vi "_unitOperForRS232_EEPROM_vna_jet.vi"(0 "Operations":string(combo)="read data", 1 "Data to write":u8[](array[numeric])=[46, 46, 46, 46, 46, 46, 46, 76, 117, 120, 115, 104, 97, 114, 101, 32, 83, 90, 32, 32, 32, 32, 32, 32, 0, 0, 9, 58, 88, 88, 88, 88, 88, 45, 88, 88, 88, 88, 32, 32, 32, 32, 32, 32, 69, 32, 32, 32, 0, 0, 0, 0, 0, 56, 56, 56, 56, 56, 56, 56, 56, 56, 56, 32, 32, 32, 32, 32, 32, 48, 56, 48, 51, 51, 0, 0, 0, 0, 0, 46, 46, 46, 46, 46, 46, 46, 46, 46, 46, 32, 105, 50, 99, 32, 116, 101, 115, 116, 105, 110, 103, 45, 45, 45, 45, 45, 32, 99, 111, 109, 112, 108, 101, 116, 101, 100, 32, 97, 110, 100, 32, 115, 117, 99, 99, 101, 115, 115, 102, 117, 108] format="%x", 3 "StartByte":i32 format="%.0x", 6 "Steps":string[](array[string])=["modify byte 127", "read byte 0 to 127", "read byte 128 to 255"], 7 "W&RDLength":i32=86, 12 "Auto":bool=TRUE) -> (15 "random_array":i32[](array[numeric])=[255, 255, 0, 0, 0, 0, 0, 0, 0, 0, 0, 0, 0, 0, 0, 0, 0, 0, 0, 0, 0, 0, 0, 0, 0, 0, 0, 0, 0, 0, 0, 0] format="%.0x", 17 "Message":string="Read EEPROM", 19 "R A I 128 to 255":u8[](array[numeric])=[3, 4, 33, 1, 0, 0, 4, 65, 132, 128, 213, 0, 103, 0, 0, 0, 0, 0, 1, 0, 72, 73, 83, 69, 84, 69, 67, 0, 0, 0, 0, 0, 0, 0, 0, 0, 0, 0, 0, 0, 76, 48, 48, 84, 72, 48, 48, 50, 45, 77, 49, 45, 82, 0, 0, 0, 65, 0, 0, 0, 1, 0, 0, 250, 0, 0, 0, 0, 49, 50, 51, 50, 55, 49, 48, 48, 48, 51, 0, 0, 0, 0, 0, 0, 49, 50, 49, 49, 50, 50, 0, 0, 0, 0, 0, 28, 72, 51, 67, 0, 0, 0, 0, 0, 0, 0, 0, 48, 52, 48, 52, 65, 49, 49, 50, 1, 2, 0, 1, 0, 0, 0, 0, 0, 0, 0, 0, 95, 0, 0, 0, 0, 0, 0, 0, 0, 0, 0, 0, 0, 0, 0, 0, 0, 0, 0, 0, 0, 0, 0, 0, 0, 0, 0, 0, 0, 0, 0, 0, 0, 0, 0, 0, 0, 0, 0, 0, 0, 0, 0, 0, 0, 0, 0, 0, 0, 0, 0, 0, 0, 0, 0, 0, 0, 0, 0, 0, 0, 0, 0, 0, 0, 0, 0, 0, 0, 0, 0, 0, 0, 0, 0, 0, 0, 0, 0, 0, 0, 0, 0, 0, 0, 0, 0, 0, 0, 0, 0, 0, 0, 0, 0, 0, 0, 0, 0, 0, 0, 0, 0, 0, 0, 0, 0, 0, 0, 0, 0, 0, 0, 0, 0, 0, 0, 0, 0, 0, 0, 0, 0, 0, 0, 0, 0, 0, 0] format="%x")   [LabVIEW 2011]
panel:
  in  "Commands_input":string[](array[string])
  out "rad_num":string
  out "EndByte":i32=86
  out "RD A 128 to 255":string[][](array[string])
  out "RD 128 to 255":string
  in  "WData size":u32=1
  out "Result":bool=TRUE
  out "VISA resource":refnum<visa-resource-name>="COM1"
  out "error out":errorcluster={"status"=FALSE, "code"=1073676294, "source"="RS232-I2C-EEPROM.vi中的VISA读取"}
  in  "VISA resource name":refnum<visa-resource-name>="COM1"
  in  "Select channel":u32 max=1
  in  "Mode":u32(ring) items=["0~EasyI2C", "1~TimingI2C"]
  # "1"
  # "2"
  # "3"
  # "序号       0 to 127  128 to 255"
  # "0 to 127  128 to 255"
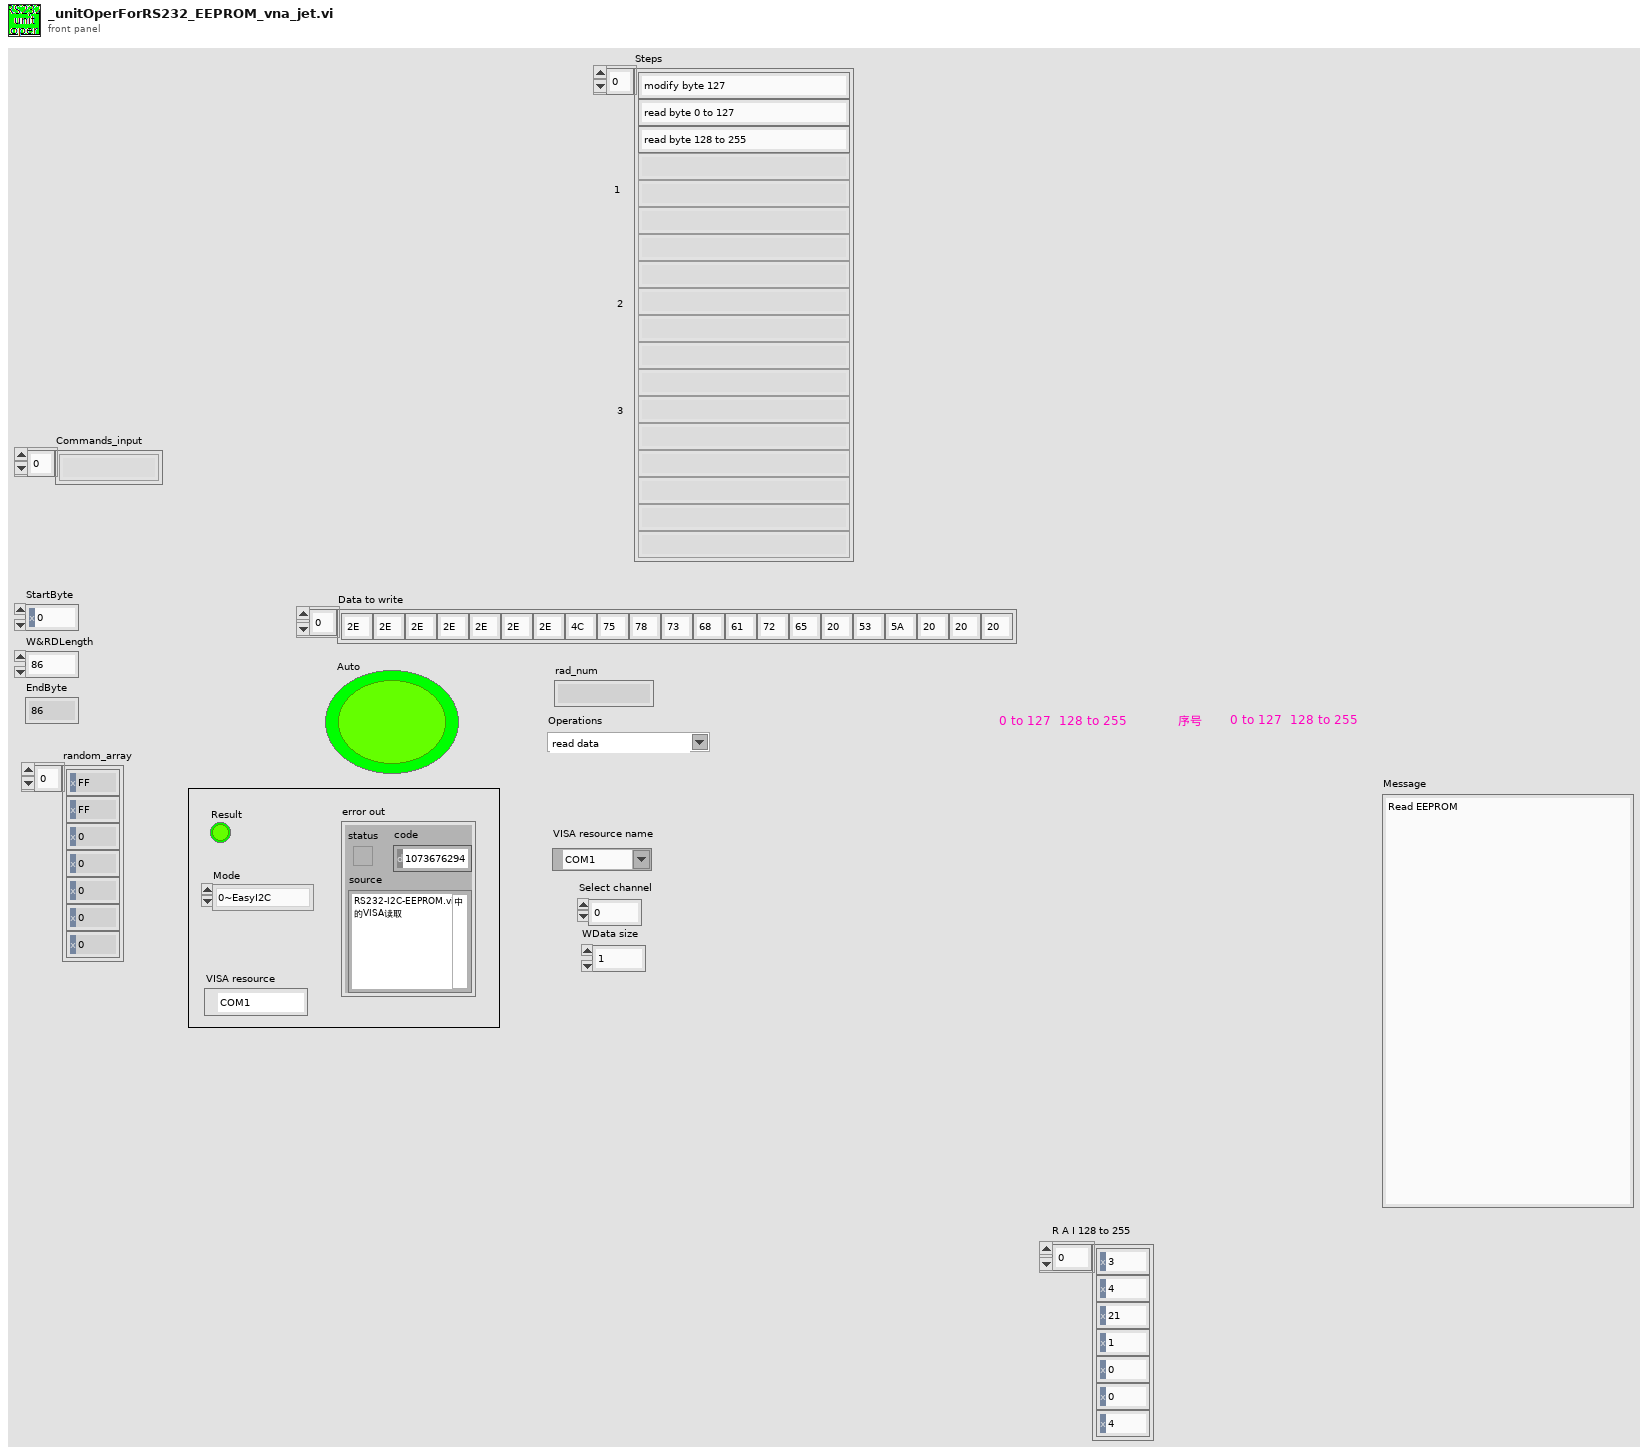
[diagram p1: front panel]
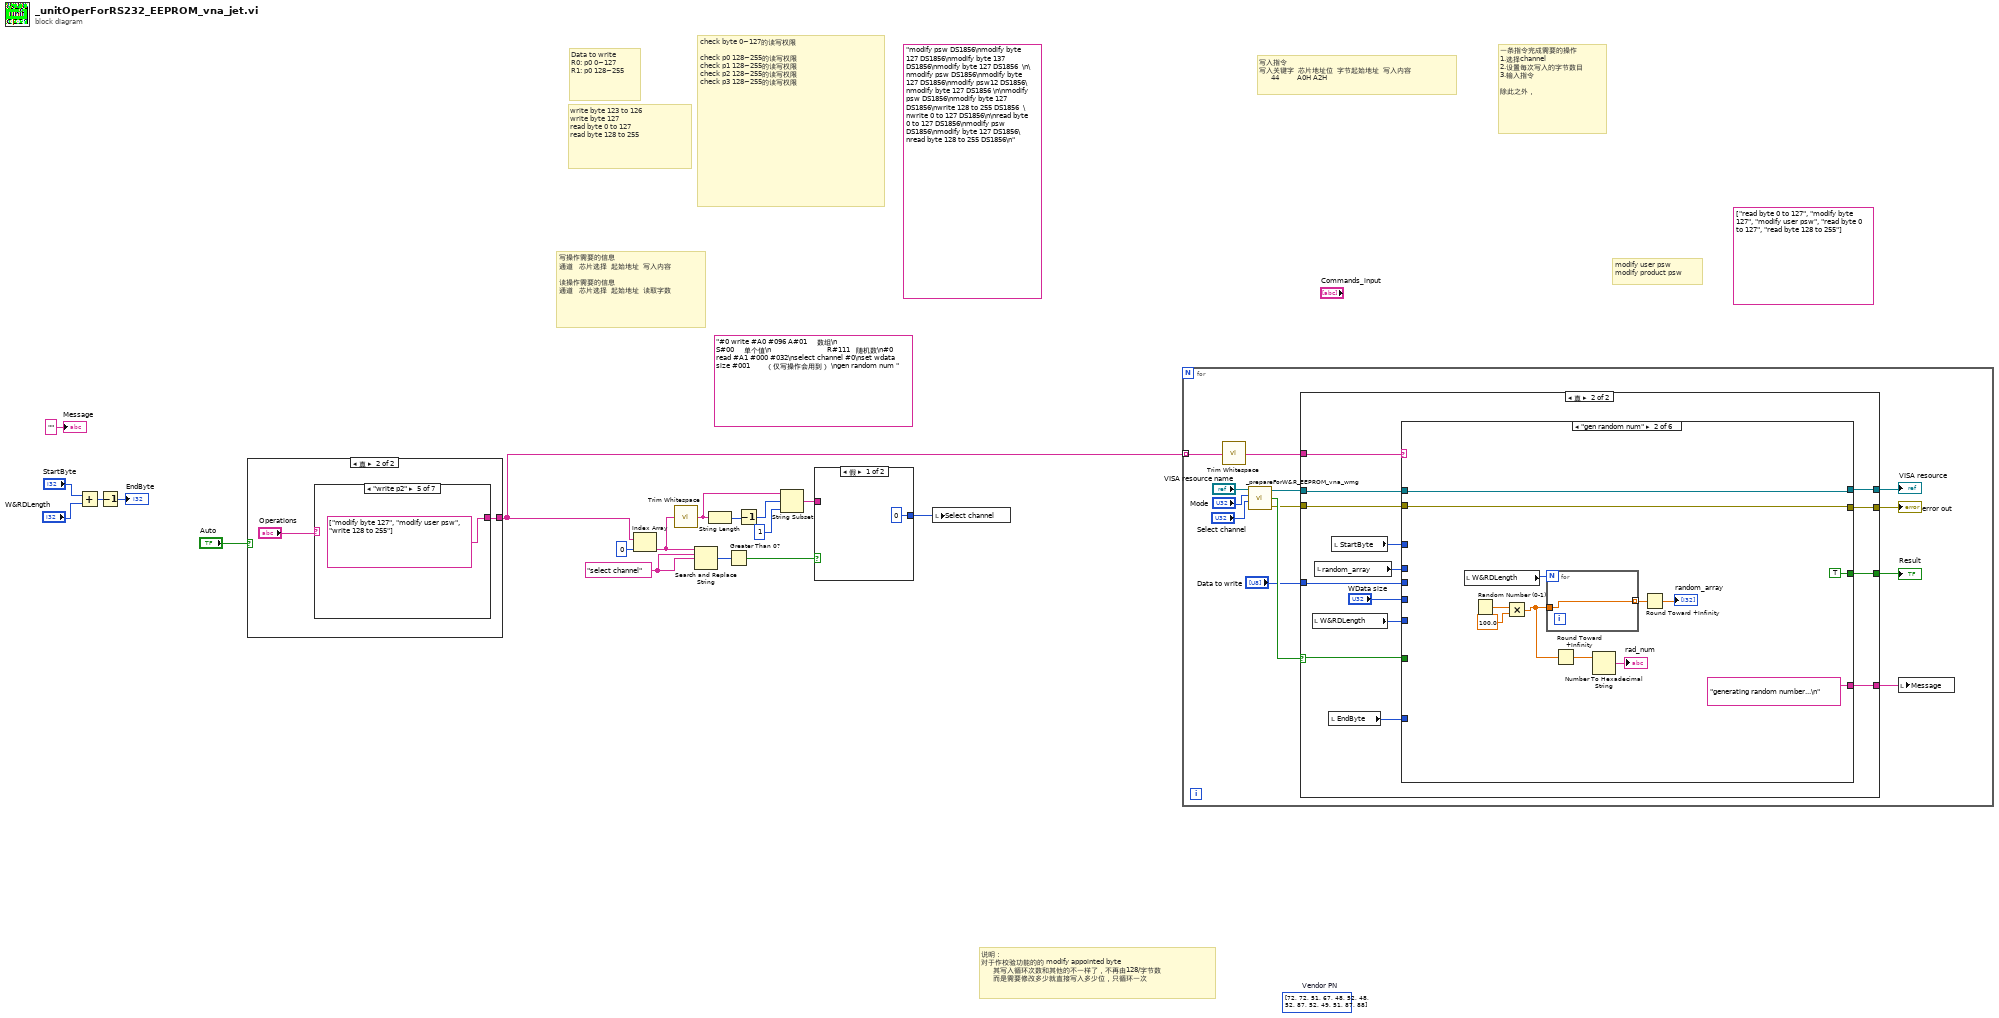
[diagram p0: block diagram]
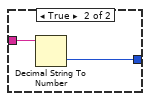
[diagram p2: hidden frame]
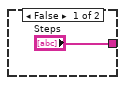
[diagram p3: hidden frame]
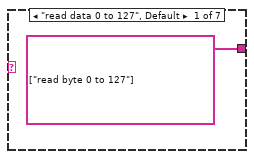
[diagram p4: hidden frame]
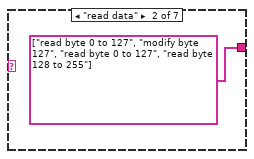
[diagram p5: hidden frame]
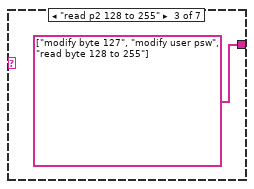
[diagram p6: hidden frame]
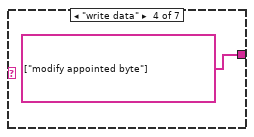
[diagram p7: hidden frame]
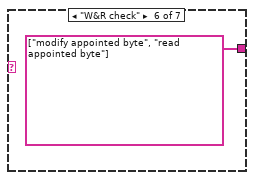
[diagram p8: hidden frame]
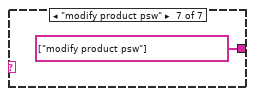
[diagram p9: hidden frame]
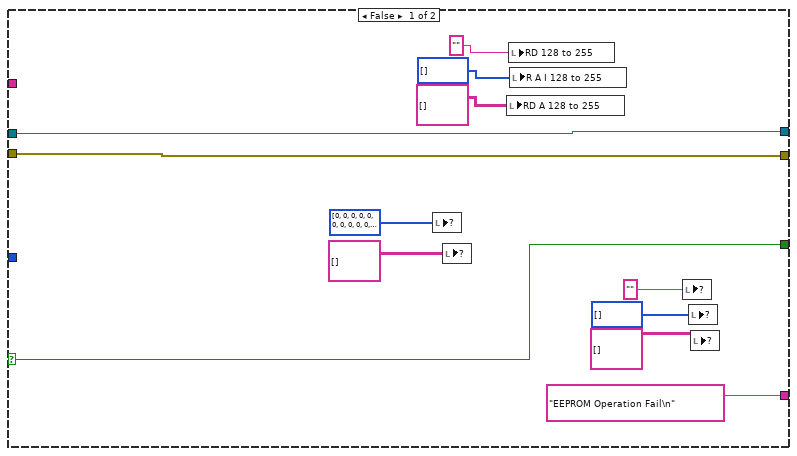
[diagram p10: hidden frame]
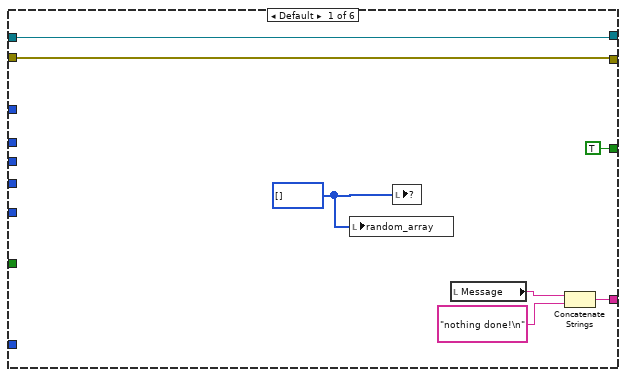
[diagram p11: hidden frame]
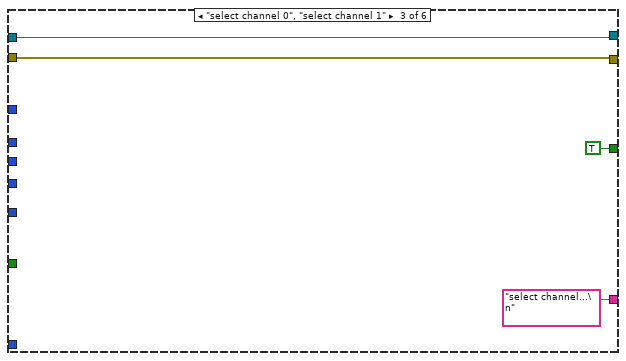
[diagram p12: hidden frame]
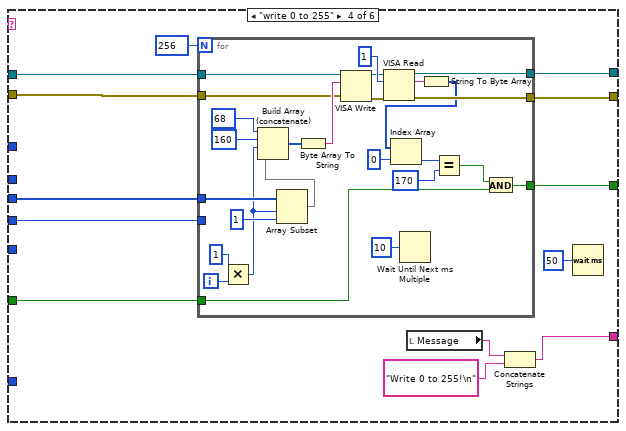
[diagram p13: hidden frame]
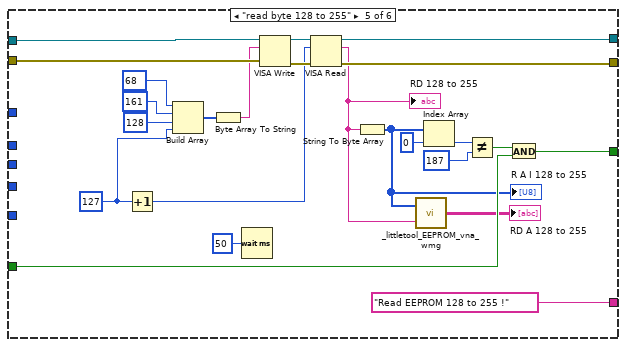
[diagram p14: hidden frame]
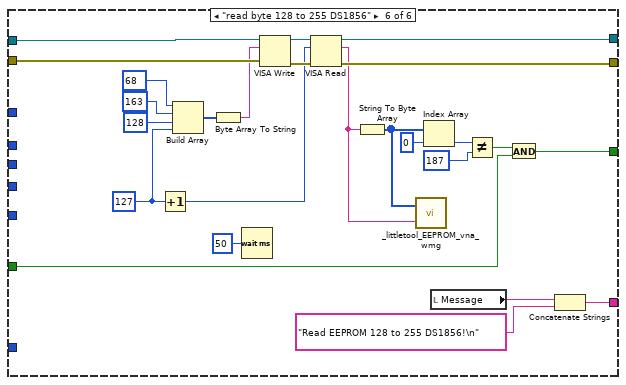
[diagram p15: hidden frame]
diagram:
  w10 = "select channel" ("搜索字符串")
  (unwired) i32[] [72, 72, 51, 67, 48, 52, 48, 52, 87, 52, 49, 51, 87, 88]  # Vendor PN
  (unwired) string[] ["read byte 0 to 127", "modify byte 127", "modify user psw", "read byte 0 to 127", "read byte 128 to 255"]
  (unwired) "#0 write #A0 #096 A#01     数组\n                            S#00     单个值\n                            R#111   随机数\n#0 read #A1 #000 #032\nselect channel #0\nset wdata size #001        （仅写操作会用到） \ngen random num "
  (unwired) "modify psw DS1856\nmodify byte 127 DS1856\nmodify byte 137 DS1856\nmodify byte 127 DS1856  \n\nmodify psw DS1856\nmodify byte 127 DS1856\nmodify psw12 DS1856\nmodify byte 127 DS1856 \n\nmodify psw DS1856\nmodify byte 127 DS1856\nwrite 128 to 255 DS1856  \nwrite 0 to 127 DS1856\n\nread byte 0 to 127 DS1856\nmodify psw DS1856\nmodify byte 127 DS1856\nread byte 128 to 255 DS1856\n"
  # "说明：\n对于作校验功能的的 modify appointed byte\n      其写入循环次数和其他的不一样了，不再由128/字节数\n      而是需要修改多少就直接写入多少位，只循环一次"
  # "写操作需要的信息\n通道   芯片选择  起始地址  写入内容\n\n读操作需要的信息\n通道   芯片选择  起始地址  读取字数"
  # "一条指令完成需要的操作\n1.选择channel\n2.设置每次写入的字节数目\n3.输入指令\n\n除此之外，"
  # "写入指令\n写入关键字  芯片地址位  字节起始地址  写入内容\n      44         A0H A2H"
  # "modify user psw\nmodify product psw"
  # "check byte 0~127的读写权限\n      \ncheck p0 128~255的读写权限\ncheck p1 128~255的读写权限\ncheck p2 128~255的读写权限\ncheck p3 128~255的读写权限"
  # "Data to write\nR0: p0 0~127\nR1: p0 128~255"
  # "write byte 123 to 126\nwrite byte 127\nread byte 0 to 127\nread byte 128 to 255"
  n1 = Add(x="StartByte", y="W&RDLength") -> (x+y=w14:i32)
  n2 = Decrement(x=w14) -> (x-1=→"EndByte":i32)
  n3 = case shown="真" "Auto" {
    tunnel: ["Steps" w21] -> w18
    frame False {
    }
    frame True {
      n4 = case shown="\"write p2\"" "Operations" {
        tunnel: [string[] ["read byte 0 to 127"] string[] ["read byte 0 to 127", "modify byte 127", "read byte 0 to 127", "read byte 128 to 255"] string[] ["modify byte 127", "modify user psw", "read byte 128 to 255"] string[] ["modify appointed byte"] string[] ["modify byte 127", "modify user psw", "write 128 to 255"] string[] ["modify appointed byte", "read appointed byte"] string[] ["modify product psw"]] -> w21
        frame "read data 0 to 127", Default {
        }
        frame "read data" {
        }
        frame "read p2 128 to 255" {
        }
        frame "write data" {
        }
        frame "write p2" {
        }
        frame "W&R check" {
        }
        frame "modify product psw" {
        }
      }
    }
  }
  n5 = Index Array(array=w18, index=0 ("索引")) -> (element=w7:string)
  n6 = call <vilib>:"Trim Whitespace.vi"("string"=w7) -> ("trimmed string"=w6:string)  [unwired: 1 in]
  n7 = Search and Replace String(input string=w7, search string=w10, replace string=w10) -> (number of replacements=w9:i32)  [unwired: 5 in, 3 out]
  n8 = String Length(string=w6) -> (length=w5:i32)
  n9 = Greater Than 0?(x=w9) -> (x > 0?=w8:bool)
  n10 = Decrement(x=w5) -> (x-1=w4:i32)
  n11 = String Subset(string=w6, offset (0)=w4, length (rest)=1 ("长度（剩余）")) -> (substring=w2:string)
  n12 = case shown="假" w8 {
    tunnel: w2 -> [_ w31]
    tunnel: [0 w30] -> w1
    frame False {
    }
    frame True {
      n13 = Decimal String To Number(string=w31) -> (number=w30:i32)  [unwired: 2 in, 1 out]
    }
  }
  n14 = local write "Select channel"(w1) -> ()
  n15 = for {
    tunnel: w18 -> [w33] mode=indexing
    n16 = call <vilib>:"Trim Whitespace.vi"("string"=w33) -> ("trimmed string"=w32:string)  [unwired: 1 in]
    n17 = call "_prepareForW&R_EEPROM_vna_wmg.vi"("Select channel"="Select channel", "Mode"="Mode", "VISA resource name"="VISA resource name") -> ("错误输出"=w41:errorcluster, "x = y?"=w44:bool, "VISA资源名称输出"=w43:refnum<visa-resource-name>)  [unwired: 1 in]
    n18 = case shown="真" w44 {
      selector: w44 -> [w53 w65]
      tunnel: w43 -> [w55 w70]
      tunnel: w41 -> [w56 w69]
      tunnel: w32 -> [_ w68]
      tunnel: "Data to write" -> [_ w67]
      tunnel: [w56 w64] -> w36
      tunnel: [w55 w63] -> w37
      tunnel: ["EEPROM Operation Fail\n" ("message") w62] -> w35
      tunnel: [w53 w61] -> w34
      frame False {
        n19 = local write item#-1(i32[] [0, 0, 0, 0, 0, 0, 0, 0, 0, 0, 0, 0, 0, 0, 0, 0, 0, 0, 0, 0, 0, 0, 0, 0, 0, 0, 0, 0, 0, 0, 0, 0, 0, 0, 0, 0, 0, 0, 0, 0, 0, 0, 0, 0, 0, 0, 0, 0, 0, 0, 0, 0, 0, 0, 0, 0, 0, 0, 0, 0, 0, 0, 0, 0, 0, 0, 0, 0, 0, 0, 0, 0, 0, 0, 0, 0, 0, 0, 0, 0, 0, 0, 0, 0, 0, 0, 0, 0, 0, 0, 0, 0, 0, 0, 0, 0, 0, 0, 0, 0, 0, 0, 0, 0, 0, 0, 0, 0, 0, 0, 0, 0, 0, 0, 0, 0, 0, 0, 0, 0, 0, 0, 0, 0, 0, 0, 0, 0, 0, 0, 0, 0, 0, 0, 0, 0, 0, 0, 0, 0, 0, 0, 0, 0, 0, 0, 0, 0, 0, 0, 0, 0, 0, 0, 0, 0, 0, 0, 0, 0, 0, 0, 0, 0, 0, 0, 0, 0, 0, 0, 0, 0, 0, 0, 0, 0, 0, 0, 0, 0, 0, 0, 0, 0, 0, 0, 0, 0, 0, 0, 0, 0, 0, 0, 0, 0, 0, 0, 0, 0, 0, 0, 0, 0, 0, 0, 0, 0, 0, 0, 0, 0, 0, 0, 0, 0, 0, 0, 0, 0, 0, 0, 0, 0, 0, 0, 0, 0, 0, 0, 0, 0, 0, 0, 0, 0, 0, 0, 0, 0, 0, 0, 0, 0, 0, 0, 0, 0, 0, 0, 0, 0, 0, 0, 0, 0] ("Data from Read")) -> ()
        n20 = local write item#-1(string[][] [] ("EEPROM read data")) -> ()
        n21 = local write "RD A 128 to 255"(string[][] [] ("R A C 0 to 127")) -> ()
        n22 = local write "RD 128 to 255"("") -> ()
        n23 = local write "R A I 128 to 255"(u8[] [] ("R A I 0 to 127")) -> ()
        n24 = local write item#-1("") -> ()
        n25 = local write item#-1(u8[] [] ("R A I 0 to 127")) -> ()
        n26 = local write item#-1(string[][] [] ("R A C 0 to 127")) -> ()
      }
      frame True {
        n27 = local read "W&RDLength"() -> (w58:i32)
        n28 = local read "random_array"() -> (w59:i32[])
        n29 = local read "EndByte"() -> (w57:i32)
        n30 = local read "StartByte"() -> (w60:i32)
        n31 = case shown="\"gen random num\"" w68 {
          tunnel: w70 -> [w77 w88 w94 w107 w157 w182]
          tunnel: w69 -> [w75 w87 w93 w106 w156 w181]
          tunnel: w67 -> [_ _ _ w100 _ _]
          tunnel: [w77 w88 w94 w103 w151 w176] -> w63
          tunnel: [w75 w87 w93 w105 w150 w175] -> w64
          tunnel: "WData size" -> [_ _ _ w104 _ _]
          tunnel: w65 -> [_ _ _ w102 w145 w171]
          tunnel: [w73 "generating random number...\n" ("Message") "select channel...\n" ("Message") w95 "Read EEPROM 128 to 255 !" ("Message") w161] -> w62
          tunnel: [TRUE TRUE TRUE w101 w143 w169] -> w61
          tunnel: w60 -> [_ _ _ _ _ _]
          tunnel: w59 -> [_ _ _ _ _ _]
          tunnel: w58 -> [_ _ _ _ _ _]
          tunnel: w57 -> [_ _ _ _ _ _]
          frame Default {
            w74 = i32[] []
            n32 = local write "random_array"(w74) -> ()
            n33 = local write item#-1(w74) -> ()
            n34 = local read "Message"() -> (w72:string)
            n35 = Concatenate Strings(w72, "nothing done!\n" ("Message")) -> (w73:string)
          }
          frame "gen random num" {
            n36 = local read "W&RDLength"() -> (w85:i32)
            n37 = Random Number (0-1)() -> (number: 0 to 1=w81:dbl)
            n38 = Multiply(x=w81, y=100.0) -> (x*y=w80:dbl)
            n39 = for {
              N: w85 -> [_]
              tunnel: [w90] -> w84 mode=indexing
              tunnel: w80 -> [w90]
            }
            n40 = Round Toward +Infinity(x=w80) -> (ceil(x): smallest int >= x=w79:dbl)
            n41 = Number To Hexadecimal String(2:w79) -> (0:→"rad_num":string)  [unwired: 1 in]
            n42 = Round Toward +Infinity(x=w84) -> (ceil(x): smallest int >= x=→"random_array":dbl[])
          }
          frame "select channel 0", "select channel 1" {
          }
          frame "write 0 to 255" {
            n43 = for {
              N: 256 -> [_]
              tunnel: w107 -> [w129]
              tunnel: w100 -> [w111]
              tunnel: w106 -> [w127]
              tunnel: [w122] -> w105
              tunnel: w104 -> [_]
              tunnel: [w120] -> w103
              tunnel: w102 -> [w115]
              tunnel: [w114] -> w101
              i -> [w113]
              n44 = Multiply(x=1, y=w113) -> (x*y=w109:i32)
              n45 = Array Subset(array=w111, index=w109, length=1 ("长度")) -> (w108:u8[])
              n46 = Build Array (concatenate)(u32 68 ("Write data"), u32 160 ("size (0)"), w109, w108) -> (w132:u32[])
              n47 = Byte Array To String(unsigned byte array=w132) -> (string=w130:string)
              n48 = VISA Write(VISA resource name=w129, write buffer=w130, error in (no error)=w127) -> (VISA resource name out=w123:refnum<visa-resource-name>, error out=w121:errorcluster)  [unwired: 1 out]
              n49 = VISA Read(VISA resource name=w123, byte count=u32 1, error in (no error)=w121) -> (VISA resource name out=w120:refnum<visa-resource-name>, read buffer=w119:string, error out=w122:errorcluster)  [unwired: 1 out]
              n50 = Wait Until Next ms Multiple(millisecond multiple=u32 10) -> ()  [unwired: 1 out]
              n51 = String To Byte Array(string=w119) -> (unsigned byte array=w118:u8[])
              n52 = Index Array(array=w118, index=0) -> (element=w117:u8)
              n53 = Equal?(x=w117, y=u32 170 ("size (0)")) -> (x = y?=w116:bool)
              n54 = And(x=w116, y=w115) -> (x .and. y?=w114:bool)
            }
            n55 = local read "Message"() -> (w97:string)
            n56 = Concatenate Strings(w97, "Write 0 to 255!\n" ("Message")) -> (w95:string)
            n57 = Wait (ms)(milliseconds to wait=u32 50 ("等待时间（毫秒）")) -> ()  [unwired: 1 out]
          }
          frame "read byte 128 to 255" {
            w134 = u32 127 ("size (0)")
            n58 = Increment(x=w134) -> (x+1=w136:u32)
            n59 = Build Array(u32 68 ("Read data"), u32 161 ("size (0)"), u32 128 ("size (0)"), w134) -> (w155:u32[])
            n60 = Byte Array To String(unsigned byte array=w155) -> (string=w154:string)
            n61 = Wait (ms)(milliseconds to wait=u32 50 ("等待时间（毫秒）")) -> ()  [unwired: 1 out]
            n62 = VISA Write(VISA resource name=w157, write buffer=w154, error in (no error)=w156) -> (VISA resource name out=w153:refnum<visa-resource-name>, error out=w152:errorcluster)  [unwired: 1 out]
            n63 = VISA Read(VISA resource name=w153, byte count=w136, error in (no error)=w152) -> (VISA resource name out=w151:refnum<visa-resource-name>, read buffer=w139:string, error out=w150:errorcluster)  [unwired: 1 out]
            "RD 128 to 255" <- w139
            n64 = String To Byte Array(string=w139) -> (unsigned byte array=w137:u8[])
            "R A I 128 to 255" <- w137
            n65 = call "_littletool_EEPROM_vna_wmg.vi"("read buffer"=w139, "inputArray"=w137) -> ("数组"=→"RD A 128 to 255":string[][])
            n66 = Index Array(array=w137, index=0) -> (element=w146:u8)
            n67 = Not Equal?(x=w146, y=u32 187 ("size (0)")) -> (x != y?=w144:bool)
            n68 = And(x=w144, y=w145) -> (x .and. y?=w143:bool)
          }
          frame "read byte 128 to 255 DS1856" {
            w158 = u32 127 ("size (0)")
            n69 = Increment(x=w158) -> (x+1=w165:u32)
            n70 = Build Array(u32 68 ("Read data"), u32 163 ("size (0)"), u32 128 ("size (0)"), w158) -> (w180:u32[])
            n71 = Byte Array To String(unsigned byte array=w180) -> (string=w179:string)
            n72 = Wait (ms)(milliseconds to wait=u32 50 ("等待时间（毫秒）")) -> ()  [unwired: 1 out]
            n73 = VISA Write(VISA resource name=w182, write buffer=w179, error in (no error)=w181) -> (VISA resource name out=w178:refnum<visa-resource-name>, error out=w177:errorcluster)  [unwired: 1 out]
            n74 = VISA Read(VISA resource name=w178, byte count=w165, error in (no error)=w177) -> (VISA resource name out=w176:refnum<visa-resource-name>, read buffer=w163:string, error out=w175:errorcluster)  [unwired: 1 out]
            n75 = String To Byte Array(string=w163) -> (unsigned byte array=w162:u8[])
            n76 = call "_littletool_EEPROM_vna_wmg.vi"("read buffer"=w163, "inputArray"=w162) -> ()  [unwired: 1 out]
            n77 = Index Array(array=w162, index=0) -> (element=w172:u8)
            n78 = local read "Message"() -> (w160:string)
            n79 = Not Equal?(x=w172, y=u32 187 ("size (0)")) -> (x != y?=w170:bool)
            n80 = And(x=w170, y=w171) -> (x .and. y?=w169:bool)
            n81 = Concatenate Strings(w160, "Read EEPROM 128 to 255 DS1856!\n" ("Message")) -> (w161:string)
          }
        }
      }
    }
    "Result" <- w34
    "VISA resource" <- w37
    "error out" <- w36
    n82 = local write "Message"(w35) -> ()
  }
  "Message" <- "" ("Message")
